vi "SortArraysPLC.vi"(9 "Pop-up Con.":refnum<vi>[](array[refnum]), 11 "FPIndicator in":refnum<vi>[](array[refnum]), 13 "DIMControlMon":refnum<vi>[](array[refnum]), 15 "DIMControSet":refnum<vi>[](array[refnum]), 17 "SetValueInfo":refnum<vi>[](array[refnum])) -> (8 "Pop-up Con. out":refnum<vi>[](array[refnum]), 10 "FPIndicator out":refnum<vi>[](array[refnum]), 12 "DIMControlMon out":refnum<vi>[](array[refnum]), 14 "DIMControSet out":refnum<vi>[](array[refnum]), 16 "SetValueInfo out":refnum<vi>[](array[refnum]))   [LabVIEW 2014, in "Panels.lvlib"]
uses:
  Panels.lvlib
panel:
  out "SetValueInfo Array out":string[](array[string])
  out "DIMControSet Array out":string[](array[string])
  out "DIMControlMon Array out":string[](array[string])
  out "FPIndicator Array out":string[](array[string])
  out "Pop-up Con. Array out":string[](array[string])
  out "SetValueInfo Array":string[](array[string])
  out "DIMControSet Array":string[](array[string])
  out "DIMControlMon Array":string[](array[string])
  out "FPIndicator Array":string[](array[string])
  out "Pop-up Con. Array":string[](array[string])
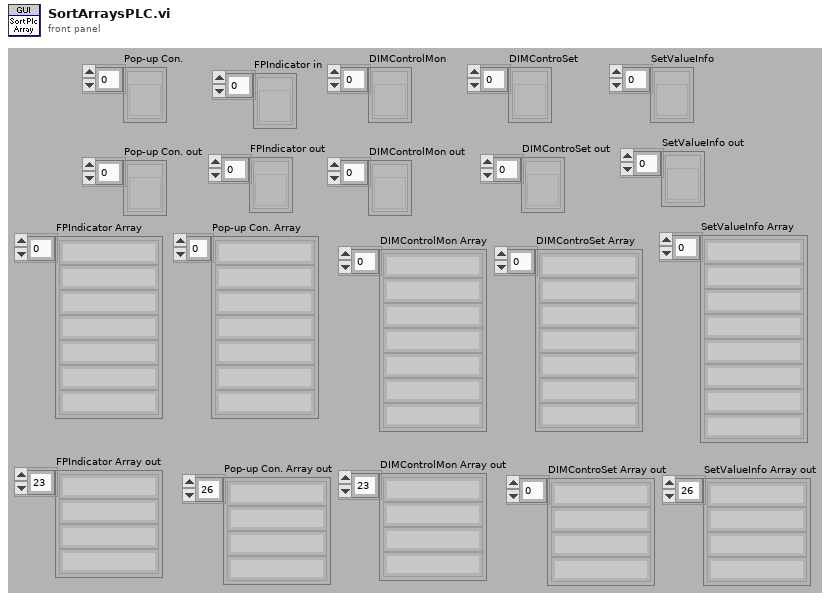
[diagram p1: front panel]
types:
  T1 = enum16{"Boolean", "DigitalNumeric", "DIM-Double", "DIM-Double-Array", "DIM-Short"}
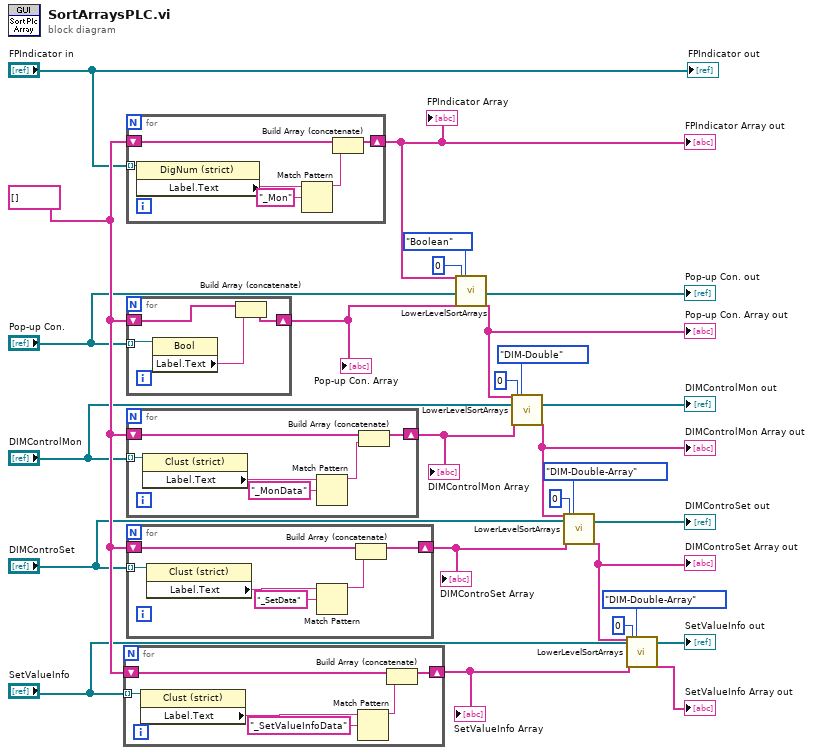
[diagram p0: block diagram]
diagram:
  w27 = string[] []
  n1 = for {
    tunnel: "SetValueInfo" -> [w31] mode=indexing
    shift-right: [w28] -> w19
    shift-left: w27 -> [w29]
    n2 = property class="Clust (strict)"(reference=w31) -> ("Label.Text"=w32:string)  [unwired: 1 in, 2 out]
    n3 = Match Pattern(string=w32, regular expression="_SetValueInfoData") -> (before substring=w30:string)  [unwired: 1 in, 3 out]
    n4 = Build Array (concatenate)(w29, w30) -> (w28:string[])
  }
  "SetValueInfo Array" <- w19
  n5 = for {
    tunnel: "FPIndicator in" -> [w39] mode=indexing
    shift-right: [w34] -> w16
    shift-left: w27 -> [w35]
    n6 = property class="DigNum (strict)"(reference=w39) -> ("Label.Text"=w37:string)  [unwired: 1 in, 2 out]
    n7 = Match Pattern(string=w37, regular expression="_Mon") -> (before substring=w36:string)  [unwired: 1 in, 3 out]
    n8 = Build Array (concatenate)(w35, w36) -> (w34:string[])
  }
  "FPIndicator Array" <- w16
  "FPIndicator Array out" <- w16
  n9 = for {
    tunnel: "Pop-up Con." -> [w43] mode=indexing
    shift-right: [w41] -> w15
    shift-left: w27 -> [w40]
    n10 = property class="Bool"(reference=w43) -> ("Label.Text"=w42:string)  [unwired: 1 in, 2 out]
    n11 = Build Array (concatenate)(w40, w42) -> (w41:string[])
  }
  "Pop-up Con. Array" <- w15
  n12 = for {
    tunnel: "DIMControlMon" -> [w47] mode=indexing
    shift-right: [w44] -> w26
    shift-left: w27 -> [w45]
    n13 = property class="Clust (strict)"(reference=w47) -> ("Label.Text"=w48:string)  [unwired: 1 in, 2 out]
    n14 = Match Pattern(string=w48, regular expression="_MonData") -> (before substring=w46:string)  [unwired: 1 in, 3 out]
    n15 = Build Array (concatenate)(w45, w46) -> (w44:string[])
  }
  "DIMControlMon Array" <- w26
  n16 = for {
    tunnel: "DIMControSet" -> [w53] mode=indexing
    shift-right: [w50] -> w23
    shift-left: w27 -> [w51]
    n17 = property class="Clust (strict)"(reference=w53) -> ("Label.Text"=w54:string)  [unwired: 1 in, 2 out]
    n18 = Match Pattern(string=w54, regular expression="_SetData") -> (before substring=w52:string)  [unwired: 1 in, 3 out]
    n19 = Build Array (concatenate)(w51, w52) -> (w50:string[])
  }
  "DIMControSet Array" <- w23
  n20 = call "LowerLevelSortArrays.vi"("Sorted Array in"=w16, "Boolean"="Pop-up Con.", "Unsorted Array in"=w15, "Index"=0, "Type"=T1."Boolean") -> ("Boolean (sorted)"=→"Pop-up Con. out":refnum<vi>[], "Sorted Array out"=w12:string[])  [unwired: 16 in, 5 out]
  "Pop-up Con. Array out" <- w12
  n21 = call "LowerLevelSortArrays.vi"("Sorted Array in"=w12, "DIM-Double"="DIMControlMon", "Unsorted Array in"=w26, "Index"=0, "Type"=T1."DIM-Double") -> ("DIM-Double (sorted)"=→"DIMControlMon out":refnum<vi>[], "Sorted Array out"=w21:string[])  [unwired: 16 in, 5 out]
  "DIMControlMon Array out" <- w21
  n22 = call "LowerLevelSortArrays.vi"("Sorted Array in"=w21, "DIM-Double-Array"="DIMControSet", "Unsorted Array in"=w23, "Index"=0, "Type"=T1."DIM-Double-Array") -> ("DIM-Double-Array (sorted)"=→"DIMControSet out":refnum<vi>[], "Sorted Array out"=w20:string[])  [unwired: 16 in, 5 out]
  "DIMControSet Array out" <- w20
  n23 = call "LowerLevelSortArrays.vi"("Sorted Array in"=w20, "DIM-Double-Array"="SetValueInfo", "Unsorted Array in"=w19, "Index"=0, "Type"=T1."DIM-Double-Array") -> ("DIM-Double-Array (sorted)"=→"SetValueInfo out":refnum<vi>[], "Sorted Array out"=→"SetValueInfo Array out":string[])  [unwired: 16 in, 5 out]
  "FPIndicator out" <- "FPIndicator in"
